vi "关键参数区.vi"(11 "数组":u16[](array[numeric]) format="%04xH") -> (3 "关键参数区":T1)   [LabVIEW 2022 SP3, in "挥发酚.lvlib"]
panel:
  # "共占用56 WORD"
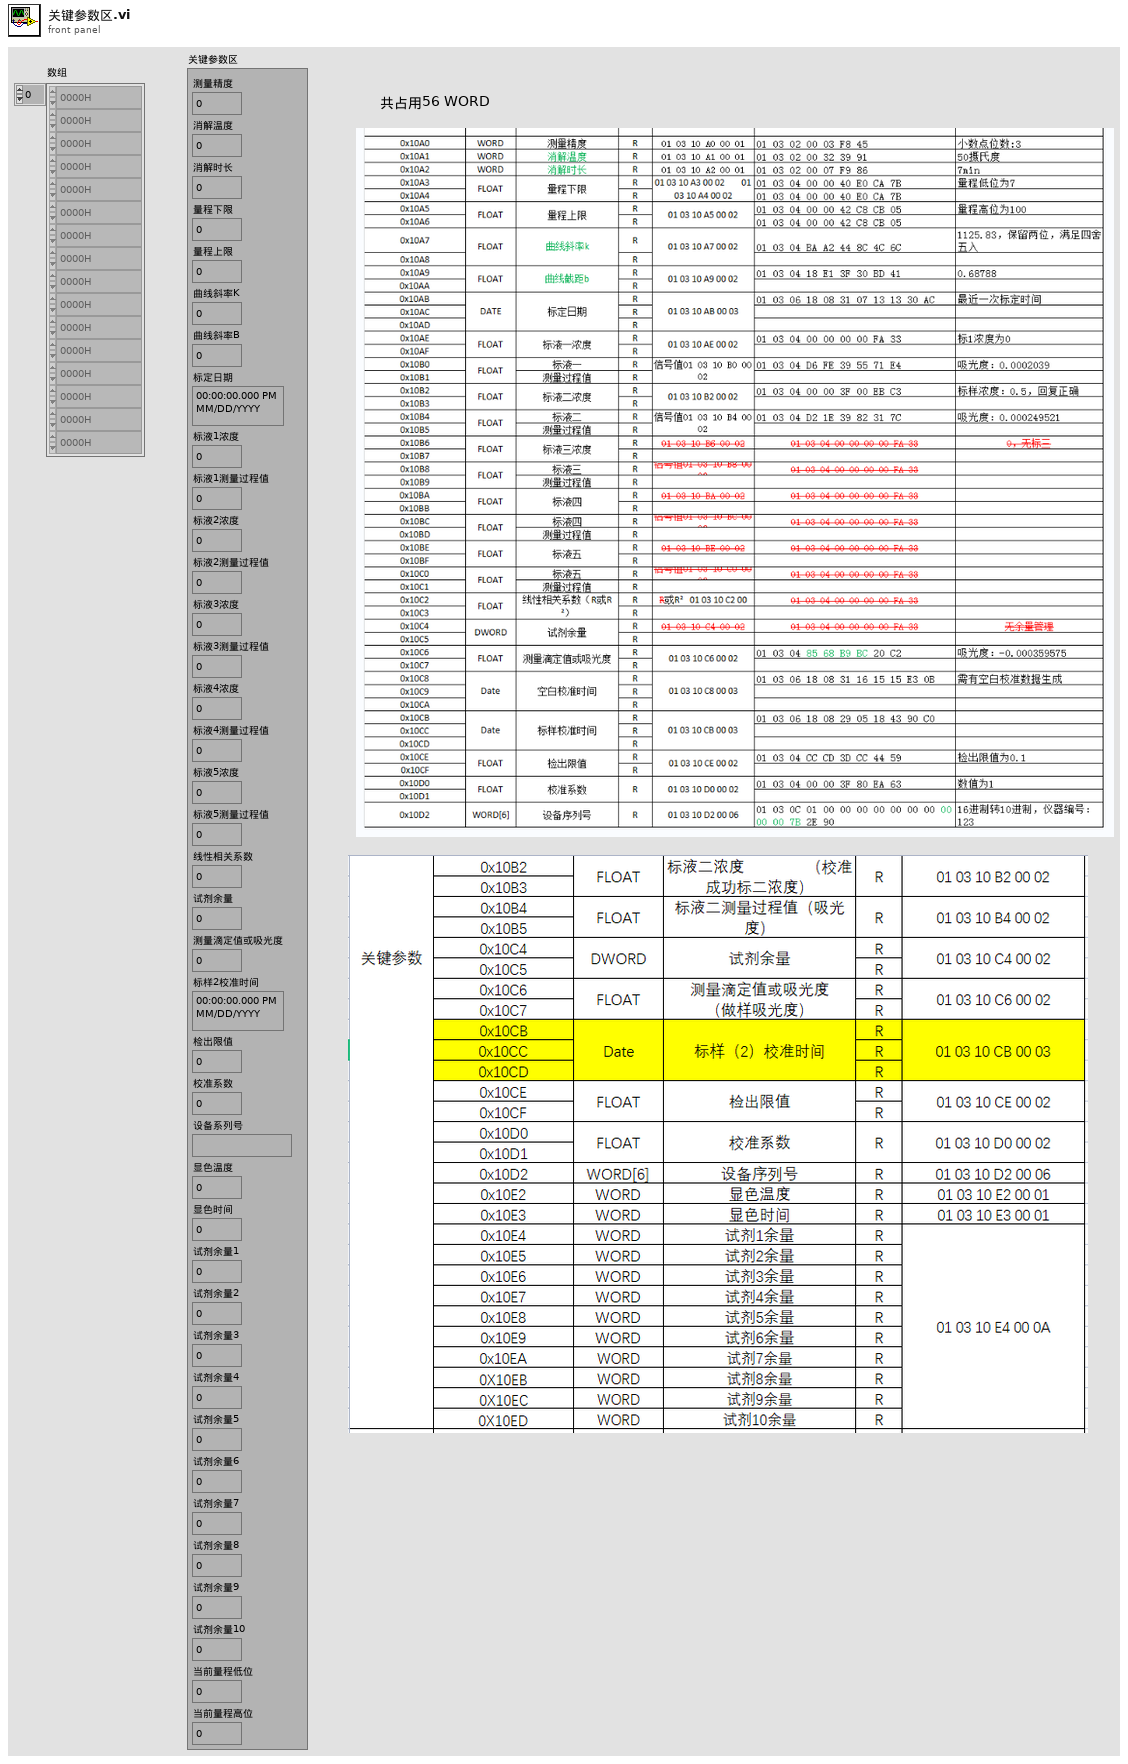
[diagram p1: front panel]
types:
  T1 = cluster{"测量精度":u16, "消解温度":u16, "消解时长":u16, "量程下限":sgl, "量程上限":sgl, "曲线斜率K":sgl, "曲线斜率B":sgl, "标定日期":timestamp, "标液1浓度":sgl, "标液1测量过程值":sgl, "标液2浓度":sgl, "标液2测量过程值":sgl, "标液3浓度":sgl, "标液3测量过程值":sgl, "标液4浓度":sgl, "标液4测量过程值":sgl, "标液5浓度":sgl, "标液5测量过程值":sgl, "线性相关系数":sgl, "试剂余量":u32, "测量滴定值或吸光度":sgl, "标样2校准时间":timestamp, "检出限值":sgl, "校准系数":sgl, "设备系列号":string, "显色温度":u16, "显色时间":u16, "试剂余量1":u16, "试剂余量2":u16, "试剂余量3":u16, "试剂余量4":u16, "试剂余量5":u16, "试剂余量6":u16, "试剂余量7":u16, "试剂余量8":u16, "试剂余量9":u16, "试剂余量10":u16, "当前量程低位":sgl, "当前量程高位":sgl}
  T2 = cluster{"WORD":u16, "WORD":u16, "WORD":u16, "FLOAT":sgl, "FLOAT":sgl, "FLOAT":sgl, "FLOAT":sgl, "time stamp":timestamp, "FLOAT":sgl, "FLOAT":sgl, "FLOAT":sgl, "FLOAT":sgl, "FLOAT":sgl, "FLOAT":sgl, "FLOAT":sgl, "FLOAT":sgl, "FLOAT":sgl, "FLOAT":sgl, "FLOAT":sgl, "WORD":u16, "FLOAT":sgl, "time stamp":timestamp, "FLOAT":sgl, "FLOAT":sgl, "string":string, "WORD":u16, "WORD":u16, "WORD":u16, "WORD":u16, "WORD":u16, "WORD":u16, "WORD":u16, "WORD":u16, "WORD":u16, "WORD":u16, "WORD":u16, "WORD":u16, "FLOAT":sgl, "FLOAT":sgl}
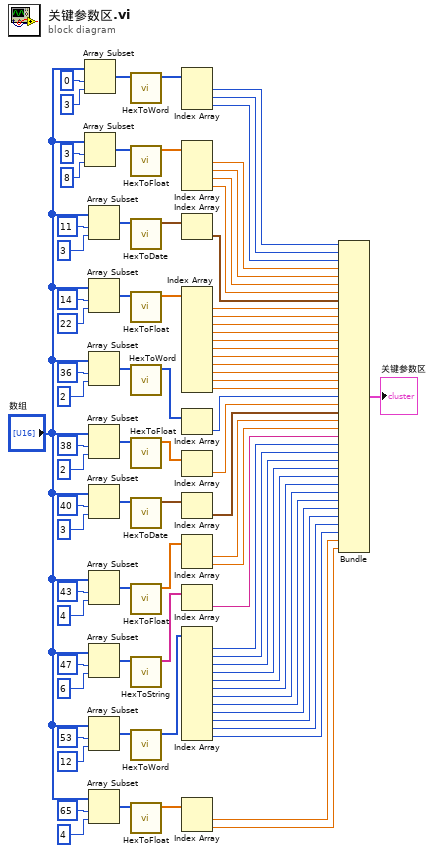
[diagram p0: block diagram]
diagram:
  n1 = Array Subset(array="数组", index=0 ("索引"), length=3 ("长度")) -> (w80:u16[])
  n2 = Array Subset(array="数组", index=3 ("索引"), length=8 ("长度")) -> (w76:u16[])
  n3 = Array Subset(array="数组", index=11 ("索引"), length=3 ("长度")) -> (w68:u16[])
  n4 = Array Subset(array="数组", index=14 ("索引"), length=22 ("长度")) -> (w63:u16[])
  n5 = Array Subset(array="数组", index=36 ("索引"), length=2 ("长度")) -> (w25:u16[])
  n6 = Array Subset(array="数组", index=38 ("索引"), length=2 ("长度")) -> (w41:u16[])
  n7 = Array Subset(array="数组", index=40 ("索引"), length=3 ("长度")) -> (w52:u16[])
  n8 = Array Subset(array="数组", index=43 ("索引"), length=4 ("长度")) -> (w48:u16[])
  n9 = Array Subset(array="数组", index=47 ("索引"), length=6 ("长度")) -> (w42:u16[])
  n10 = Array Subset(array="数组", index=53 ("索引"), length=12 ("长度")) -> (w21:u16[])
  n11 = Array Subset(array="数组", index=65 ("索引"), length=4 ("长度")) -> (w6:u16[])
  n12 = call "HexToWord.vi"("数组"=w80) -> ("WORD"=w79:u16[])  [unwired: 10 in]
  n13 = call "HexToFloat.vi"("数组"=w76) -> ("FLOAT"=w75:sgl[])  [unwired: 10 in]
  n14 = call "HexToDate.vi"("数组"=w68) -> ("DATE"=w67:timestamp[])  [unwired: 10 in]
  n15 = call "HexToFloat.vi"("数组"=w63) -> ("FLOAT"=w62:sgl[])  [unwired: 10 in]
  n16 = call "HexToWord.vi"("数组"=w25) -> ("WORD"=w24:u16[])  [unwired: 10 in]
  n17 = call "HexToFloat.vi"("数组"=w41) -> ("FLOAT"=w38:sgl[])  [unwired: 10 in]
  n18 = call "HexToDate.vi"("数组"=w52) -> ("DATE"=w51:timestamp[])  [unwired: 10 in]
  n19 = call "HexToFloat.vi"("数组"=w48) -> ("FLOAT"=w46:sgl[])  [unwired: 10 in]
  n20 = call "HexToString.vi"("数组"=w42) -> ("STRING"=w27:string[])  [unwired: 10 in]
  n21 = call "HexToWord.vi"("数组"=w21) -> ("WORD"=w20:u16[])  [unwired: 10 in]
  n22 = call "HexToFloat.vi"("数组"=w6) -> ("FLOAT"=w4:sgl[])  [unwired: 10 in]
  n23 = Index Array(array=w79) -> (element #1=w83:u16, element #2=w82:u16, element #3=w81:u16)  [unwired: 3 in]
  n24 = Index Array(array=w75) -> (element #1=w74:sgl, element #2=w73:sgl, element #3=w72:sgl, element #4=w71:sgl)  [unwired: 4 in]
  n25 = Index Array(array=w67) -> (element=w66:timestamp)  [unwired: 1 in]
  n26 = Index Array(array=w62) -> (element #1=w61:sgl, element #2=w60:sgl, element #3=w59:sgl, element #4=w58:sgl, element #5=w35:sgl, element #6=w34:sgl, element #7=w33:sgl, element #8=w32:sgl, element #9=w31:sgl, element #10=w30:sgl, element #11=w29:sgl)  [unwired: 11 in]
  n27 = Index Array(array=w24) -> (element=w55:u16)  [unwired: 1 in]
  n28 = Index Array(array=w38) -> (element=w37:sgl)  [unwired: 1 in]
  n29 = Index Array(array=w51) -> (element=w50:timestamp)  [unwired: 1 in]
  n30 = Index Array(array=w46) -> (element #1=w45:sgl, element #2=w36:sgl)  [unwired: 2 in]
  n31 = Index Array(array=w27) -> (element=w26:string)  [unwired: 1 in]
  n32 = Index Array(array=w20) -> (element #1=w19:u16, element #2=w18:u16, element #3=w17:u16, element #4=w16:u16, element #5=w15:u16, element #6=w14:u16, element #7=w13:u16, element #8=w12:u16, element #9=w11:u16, element #10=w10:u16, element #11=w9:u16, element #12=w8:u16)  [unwired: 12 in]
  n33 = Index Array(array=w4) -> (element #1=w2:sgl, element #2=w1:sgl)  [unwired: 2 in]
  n34 = Bundle("WORD"=w83, "WORD"=w82, "WORD"=w81, "FLOAT"=w74, "FLOAT"=w73, "FLOAT"=w72, "FLOAT"=w71, "time stamp"=w66, "FLOAT"=w61, "FLOAT"=w60, "FLOAT"=w59, "FLOAT"=w58, "FLOAT"=w35, "FLOAT"=w34, "FLOAT"=w33, "FLOAT"=w32, "FLOAT"=w31, "FLOAT"=w30, "FLOAT"=w29, "WORD"=w55, "FLOAT"=w37, "time stamp"=w50, "FLOAT"=w45, "FLOAT"=w36, "string"=w26, "WORD"=w19, "WORD"=w18, "WORD"=w17, "WORD"=w16, "WORD"=w15, "WORD"=w14, "WORD"=w13, "WORD"=w12, "WORD"=w11, "WORD"=w10, "WORD"=w9, "WORD"=w8, "FLOAT"=w2, "FLOAT"=w1) -> (→"关键参数区":T2)  [unwired: 1 in]
